vi "testing_continuous.vi"() -> ()   [LabVIEW 2023]
panel:
  in  "stop":bool
  in  "OK Button":bool
  out "iter_number":i32
  in  "3: stepping direction":bool=TRUE
  in  "3: AC Voltage":dbl=60.0 min=0.0 format="%.1g"
  in  "3: AC frequency":dbl=10.0 min=0.0 format="%.1f"
  out "Serial":string="ANC300B-C-2133-4009033"
  in  "ANC300 address":refnum<visa-resource-name>="COM8"
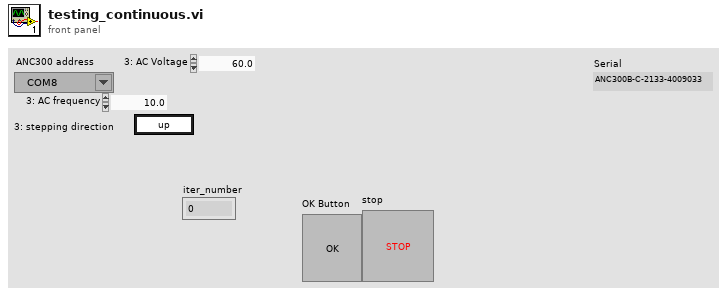
[diagram p1: front panel]
types:
  T1 = cluster{"error ":bool, "error number":i32, "error code":string}
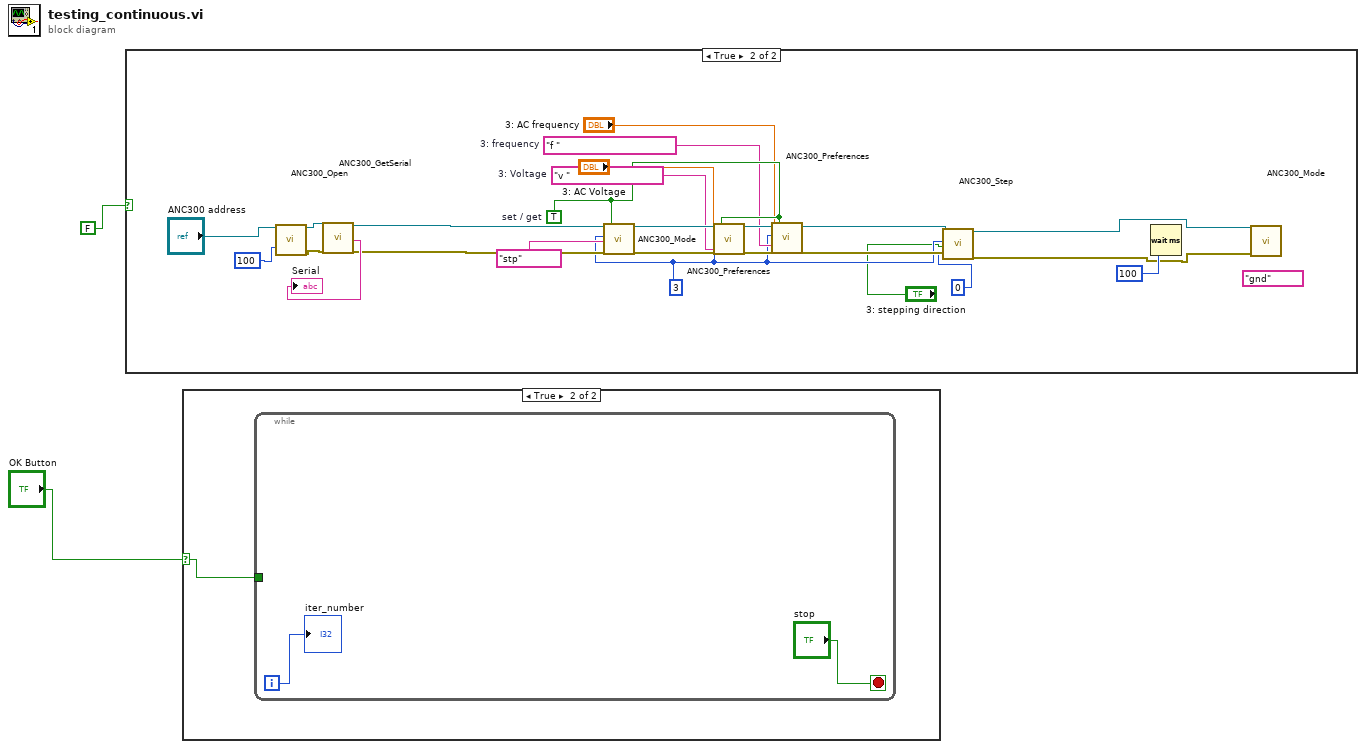
[diagram p0: block diagram]
diagram:
  n1 = case shown="True" FALSE {
    frame False {
    }
    frame True {
      (unwired) "gnd" ("3 Stepper x")
      w8 = 3
      w12 = "v "  # 3: Voltage
      w14 = "f "  # 3: frequency
      w16 = TRUE  # set / get
      n2 = call "ANC300_Open.vi"("ANC300 Communication Port In"="ANC300 address", "milliseconds to wait"=u32 100 ("millisecond timer value")) -> ("ANC300 Communication Port Out"=w26:refnum<visa-resource-name>, "error out"=w27:T1)  [unwired: 13 in, 3 out]
      n3 = call "ANC300_GetSerial.vi"("ANC300 Communication Port In"=w26, "error in"=w27) -> ("ANC300 Communication Port Out"=w9:refnum<visa-resource-name>, "Serial"=→"Serial":string, "error out"=w10:T1)  [unwired: 10 in, 5 out]
      n4 = call "ANC300_Mode.vi"("ANC300 Communication Port In"=w9, "Axis"=w8, "axis mode in"="stp", "error in"=w10, "set / get"=w16) -> ("ANC300 Communication Port Out"=w22:refnum<visa-resource-name>, "error out"=w20:T1)  [unwired: 8 in, 5 out]
      n5 = call "ANC300_Preferences.vi"("ANC300 Communication Port In"=w22, "Axis"=w8, "value in"="3: AC Voltage", "parameter"=w12, "error in"=w20, "set / get"=w16) -> ("ANC300 Communication Port Out"=w18:refnum<visa-resource-name>, "error out"=w17:T1)  [unwired: 6 in, 6 out]
      n6 = call "ANC300_Preferences.vi"("ANC300 Communication Port In"=w18, "Axis"=w8, "value in"="3: AC frequency", "parameter"=w14, "error in"=w17, "set / get"=w16) -> ("ANC300 Communication Port Out"=w21:refnum<visa-resource-name>, "error out"=w19:T1)  [unwired: 6 in, 6 out]
      n7 = call "ANC300_Step.vi"("ANC300 Communication Port In"=w21, "Axis"=w8, "stepping direction"="3: stepping direction", "number of steps [0=cont.]"=0, "error in"=w19) -> ("ANC300 Communication Port Out"=w5:refnum<visa-resource-name>, "error out"=w4:T1)  [unwired: 9 in, 4 out]
      n8 = Wait (ms)(milliseconds to wait=u32 100 ("millisecond timer value")) -> ()  [unwired: 1 out]
      n9 = call "ANC300_Mode.vi"("ANC300 Communication Port In"=w5, "error in"=w4) -> ()  [unwired: 11 in, 7 out]
    }
  }
  n10 = case shown="True" "OK Button" {
    selector: "OK Button" -> [_ w28]
    frame False {
    }
    frame True {
      n11 = while {
        tunnel: w28 -> [_]
        i -> [w30]
        stop <- "stop" stop-if-true
        "iter_number" <- w30
      }
    }
  }
